vi "UART Read Data.vi"(7 "UART #":T1=-1, 8 "error in (no error)":errorcluster, 9 "Len (LineTerm)":u8, 11 "VisaComms in":refnum<class "VisaComms.lvclass">) -> (0 "error out":errorcluster, 1 "Data":string, 3 "VisaComms out":refnum<class "VisaComms.lvclass">)   [LabVIEW 2024, in "CTI.lvlib" / "VisaComms.lvclass"]
uses:
  VisaComms.lvclass
  UART Number.ctl
  VisaComms.lvclass/VisaComms.ctl
  Clean Visa Errors.vi
  CTI.lvlib
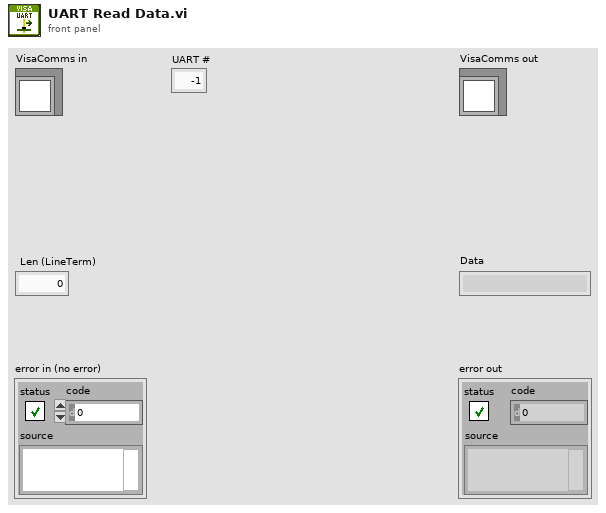
[diagram p1: front panel]
types:
  T1 = typedef "CTI.lvlib/UART Number.ctl" = i8
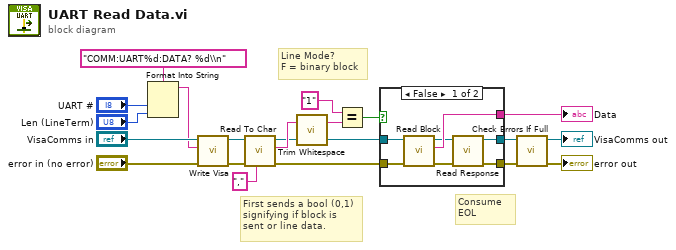
[diagram p0: block diagram]
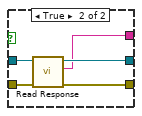
[diagram p2: hidden frame]
diagram:
  # "Line Mode?\nF = binary block"
  # "Consume EOL"
  # "First sends a bool (0,1) signifying if block is sent or line data."
  n1 = Format Into String(format string="COMM:UART%d:DATA? %d\\n", "UART #", "Len (LineTerm)") -> (resulting string=w14:string)  [unwired: 2 in, 1 out]
  n2 = call "Write Visa.vi"("error in (no error)"="error in (no error)", "write buffer"=w14, "VisaComms in"="VisaComms in") -> ("error out"=w16:errorcluster, "VisaComms out"=w12:refnum<class "VisaComms.lvclass">)  [unwired: 6 in, 1 out]
  n3 = call "Read To Char.vi"("Char"=",", "error in (no error)"=w16, "VisaComms in"=w12) -> ("error out"=w13:errorcluster, "Response"=w10:string, "VisaComms out"=w6:refnum<class "VisaComms.lvclass">)  [unwired: 6 in]
  n4 = call "Trim Whitespace.vi"("String in"=w10) -> ("Trimmed"=w9:string)  [unwired: 2 in]
  n5 = Equal?(x="1", y=w9) -> (x = y?=w5:bool)
  n6 = case shown="False" w5 {
    tunnel: w13 -> [w27 w32]
    tunnel: [w23 w31] -> w7
    tunnel: w6 -> [w25 w30]
    tunnel: [w21 w29] -> w2
    tunnel: [w24 w28] -> w4
    frame False {
      n7 = call "Read Block.vi"("error in (no error)"=w27, "VisaComms in"=w25) -> ("error out"=w26:errorcluster, "Block"=w24:string, "VisaComms out"=w22:refnum<class "VisaComms.lvclass">)  [unwired: 6 in, 1 out]
      n8 = call "Read Response.vi"("error in (no error)"=w26, "VisaComms in"=w22) -> ("error out"=w23:errorcluster, "VisaComms out"=w21:refnum<class "VisaComms.lvclass">)  [unwired: 6 in, 2 out]
    }
    frame True {
      n9 = call "Read Response.vi"("error in (no error)"=w32, "VisaComms in"=w30) -> ("error out"=w31:errorcluster, "Response"=w28:string, "VisaComms out"=w29:refnum<class "VisaComms.lvclass">)  [unwired: 6 in, 1 out]
    }
  }
  "Data" <- w4
  n10 = call "Check Errors If Full.vi"("error in (no error)"=w7, "VisaComms in"=w2) -> ("error out"=→"error out":errorcluster, "VisaComms out"=→"VisaComms out":refnum<class "VisaComms.lvclass">)  [unwired: 8 in]
